vi "Roller Button Read.vi"(8 "Button Array":bool[](array[boolean]), 9 "D-Pad":T1, 10 "Button Cluster":T3, 11 "Axes":T2) -> ()   [LabVIEW 2014]
uses:
  Real-Life Controls/D-Pad.ctl
  Common Code/Roller Mode Enum.ctl
  Auto Roller Commands.ctl
  Common Code/Change Detect Boolean.vi
  Robot Global Data.vi
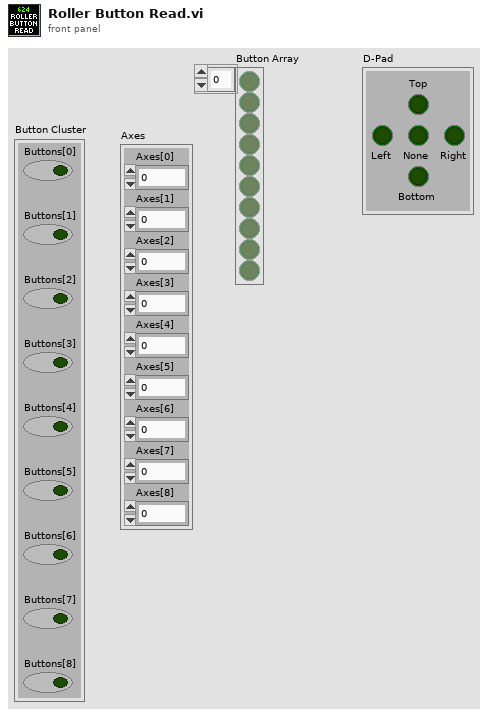
[diagram p1: front panel]
types:
  T1 = typedef "D-Pad.ctl" = cluster{"Top":bool, "Bottom":bool, "None":bool, "Right":bool, "Left":bool}
  T2 = cluster{"Axes[0]":dbl, "Axes[1]":dbl, "Axes[2]":dbl, "Axes[3]":dbl, "Axes[4]":dbl, "Axes[5]":dbl, "Axes[6]":dbl, "Axes[7]":dbl, "Axes[8]":dbl}
  T3 = cluster{"Buttons[0]":bool, "Buttons[1]":bool, "Buttons[2]":bool, "Buttons[3]":bool, "Buttons[4]":bool, "Buttons[5]":bool, "Buttons[6]":bool, "Buttons[7]":bool, "Buttons[8]":bool}
  T4 = typedef "Roller Control.ctl" = cluster{"Mode":T5, "Manual":cluster{"Manual Claw":bool, "Right Roller":bool, "Left Roller":bool, "Left Roller Back":bool, "Right Roller Back":bool}, "Left Roller Speed":dbl, "Right Roller Speed":dbl, "Left Roller Speed Back":dbl, "Right Roller Speed Back":dbl, "Auto Roller":T6}
  T5 = typedef "Roller Mode Enum.ctl" = enum16{"Manual", "Auto"}
  T6 = typedef "Auto Roller Commands.ctl" = enum16{"Grab Tote", "Idle"}
  T7 = cluster{"Manual Claw":bool, "Right Roller":bool, "Left Roller":bool, "Left Roller Back":bool, "Right Roller Back":bool}
  T8 = typedef "Roller Mode Enum.ctl" = enum16{"Manual", "Idle", "Grab Tote", "Align Tote", "Load Tote", "Unload Totes"}
  T9 = typedef "Roller Control.ctl" = cluster{"Mode":T5, "Tote Inside?":bool, "Claw Piston":bool, "Manual":cluster{"Manual Claw":bool, "Right Roller":bool, "Left Roller":bool, "Left Roller Back":bool, "Right Roller Back":bool}, "Left Roller Speed":dbl, "Right Roller Speed":dbl, "Left Roller Speed Back":dbl, "Right Roller Speed Back":dbl}
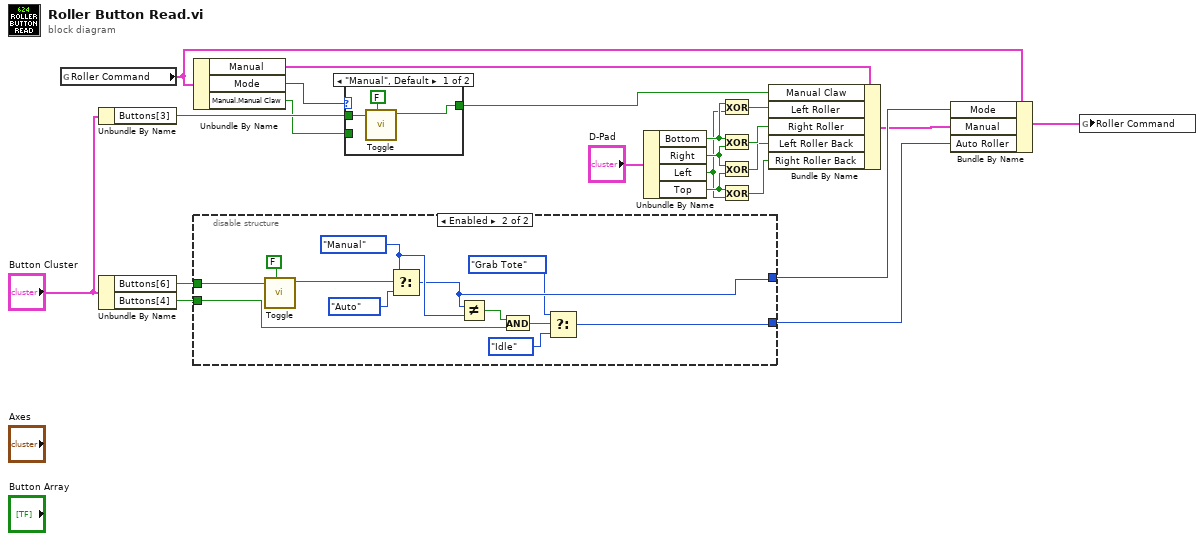
[diagram p0: block diagram]
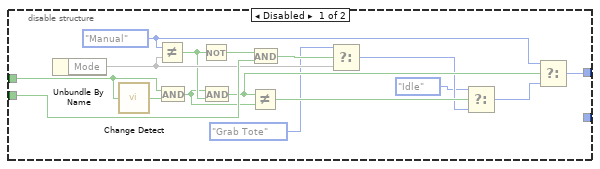
[diagram p3: hidden frame]
diagram:
  n1 = global read "Robot Global Data.vi" "Roller Command"() -> (w18:T4)
  n2 = Unbundle By Name("Button Cluster") -> ("Buttons[3]"=w5:bool)
  n3 = Unbundle By Name("Button Cluster") -> ("Buttons[6]"=w15:bool, "Buttons[4]"=w21:bool)
  n4 = Unbundle By Name(w18) -> ("Manual"=w17:T7, "Mode"=w3:T5, "Manual.Manual Claw"=w2:bool)
  n5 = disable-structure shown="Enabled" {
    disable-tunnel: w21 -> [w38 w46]
    disable-tunnel: [w36 w43] -> w20
    disable-tunnel: w15 -> [w27 w51]
    disable-tunnel: [_ w42] -> w1
    frame Disabled {
      w25 = Roller_Mode_Enum."Manual" ("Mode")
      n6 = Unbundle By Name() -> (w35:T9, "Mode"=w34)
      n7 = call-poly "Change Detect.vi"("In"=w27) -> ("Changed?"=w28:bool)
      n8 = Not Equal?(x=w25, y=w34) -> (x != y?=w33:bool)
      n9 = And(x=w27, y=w28) -> (x .and. y?=w26:bool)
      n10 = Not(x=w33) -> (.not. x?=w39:bool)
      n11 = And(x=w26, y=w33) -> (x .and. y?=w32:bool)
      n12 = Not Equal?(x=w32, y=w26) -> (x != y?=w31:bool)
      n13 = And(x=w39, y=w38) -> (x .and. y?=w37:bool)
      n14 = Select(t=Roller_Mode_Enum."Grab Tote" ("Mode"), s=w37, f=w34) -> (s? t:f=w30:T8)
      n15 = Select(t=Roller_Mode_Enum."Idle" ("s? t:f"), s=w31, f=w30) -> (s? t:f=w29:T8)
      n16 = Select(t=w25, s=w32, f=w29) -> (s? t:f=w36:u16)
    }
    frame Enabled {
      w44 = Roller_Mode_Enum."Manual" ("Mode")
      n17 = call "Toggle.vi"("Initial Value"=FALSE, "In"=w51) -> ("Toggled"=w50:bool)  [unwired: 9 in]
      n18 = Select(t=w44, s=w50, f=Roller_Mode_Enum."Auto" ("Mode")) -> (s? t:f=w43:T5)
      n19 = Not Equal?(x=w43, y=w44) -> (x != y?=w47:bool)
      n20 = And(x=w47, y=w46) -> (x .and. y?=w48:bool)
      n21 = Select(t=Auto_Roller_Commands."Grab Tote" ("Auto Roller State"), s=w48, f=Auto_Roller_Commands."Idle" ("Auto Roller State")) -> (s? t:f=w42:T6)
    }
  }
  n22 = case shown="\"Manual\", Default" w3 {
    tunnel: w5 -> [w54 _]
    tunnel: [w53 w55] -> w4
    tunnel: w2 -> [_ w55]
    frame "Manual", Default {
      n23 = call "Toggle.vi"("Initial Value"=FALSE, "In"=w54) -> ("Toggled"=w53:bool)  [unwired: 9 in]
    }
    frame "Auto" {
    }
  }
  n24 = Unbundle By Name("D-Pad") -> ("Bottom"=w8:bool, "Right"=w7:bool, "Left"=w6:bool, "Top"=w9:bool)
  n25 = Exclusive Or(1:w6, 2:w8) -> (0:w12:bool)
  n26 = Exclusive Or(1:w7, 2:w8) -> (0:w13:bool)
  n27 = Exclusive Or(1:w9, 2:w7) -> (0:w11:bool)
  n28 = Exclusive Or(1:w6, 2:w9) -> (0:w10:bool)
  n29 = Bundle By Name(cluster=w17, "Manual Claw"=w4, "Left Roller"=w12, "Right Roller"=w13, "Left Roller Back"=w11, "Right Roller Back"=w10) -> (w16:T7)
  n30 = Bundle By Name(cluster=w18, "Mode"=w20, "Manual"=w16, "Auto Roller"=w1) -> (w19:T4)
  n31 = global write "Robot Global Data.vi" "Roller Command"(w19) -> ()
